vi "Read Notify idle.vi"(8 "error in (no error)":errorcluster, 11 "BaseDriver in":refnum<class "BaseDriver.lvclass">) -> (0 "error out":errorcluster, 2 "Notify idle":bool=TRUE, 3 "BaseDriver out":refnum<class "BaseDriver.lvclass">)   [LabVIEW 2013, in "BaseDriver.lvclass"]
doc: "If Notify Idle is set to TRUE, the driver will emit messages notifying the parent application when it becomes busy (has messages to send or are waiting for acknowledgements) and when it becomes Idle (no more messages to send or receive)"
uses:
  BaseDriver.lvclass
  BaseDriver.lvclass/BaseDriver.ctl
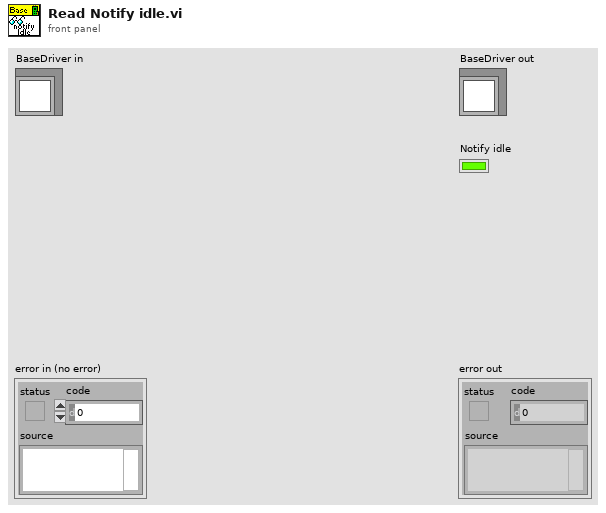
[diagram p1: front panel]
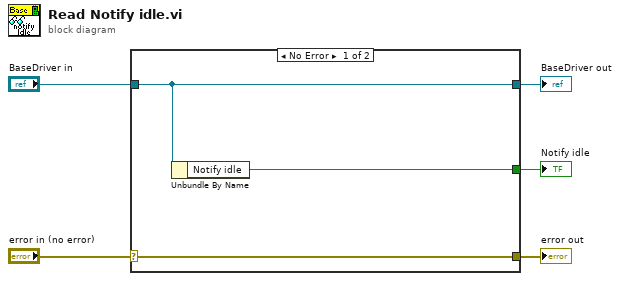
[diagram p0: block diagram]
diagram:
  n1 = case shown="No Error" "error in (no error)" {
    selector: "error in (no error)" -> [w8 w9]
    tunnel: [w8 w9] -> w4
    tunnel: [w7 w10] -> w2
    tunnel: "BaseDriver in" -> [w7 w10]
    tunnel: [w6 _] -> w1
    frame No Error {
      n2 = Unbundle By Name(w7) -> ("Notify idle"=w6:bool)
    }
    frame Error {
    }
  }
  "error out" <- w4
  "BaseDriver out" <- w2
  "Notify idle" <- w1
